vi "SetEntryJumpToMode.vi"(1 "Jump To Mode":u16(ring) items=["First", "Previous", "Next", "Last", "Item"], 3 "error in (no error)":errorcluster, 4 "Element":i16=1 min=1, 5 "VISA resource name":refnum<visa-resource-name>) -> (0 "error out":errorcluster, 2 "VISA resource name out":refnum<visa-resource-name>)   [LabVIEW 2020, in "Active Technologies AWG3000.lvlib"]
uses:
  Active Technologies AWG3000.lvlib
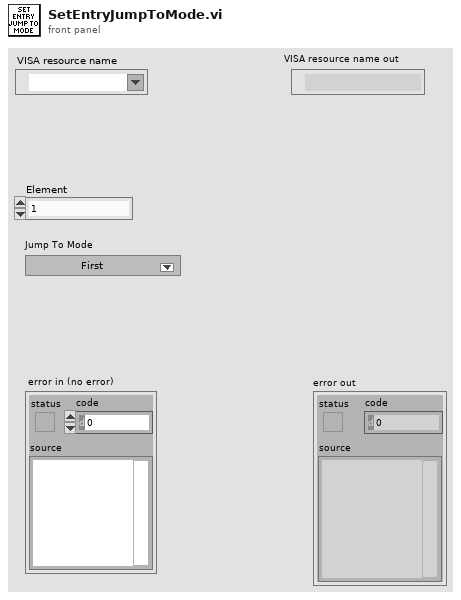
[diagram p1: front panel]
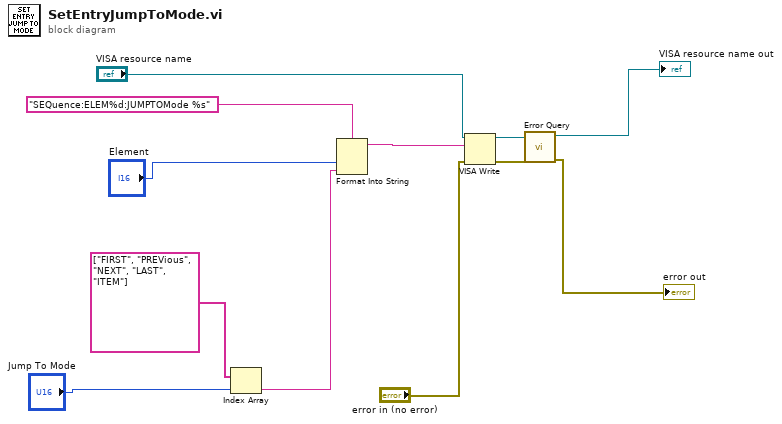
[diagram p0: block diagram]
diagram:
  n1 = Index Array(array=string[] ["FIRST", "PREVious", "NEXT", "LAST", "ITEM"], index="Jump To Mode") -> (element=w1:string)
  n2 = Format Into String(format string="SEQuence:ELEM%d:JUMPTOMode %s" ("write buffer"), "Element", w1) -> (resulting string=w4:string)  [unwired: 2 in, 1 out]
  n3 = VISA Write(VISA resource name="VISA resource name", write buffer=w4, error in (no error)="error in (no error)") -> (VISA resource name out=w9:refnum<visa-resource-name>, error out=w8:errorcluster)  [unwired: 1 out]
  n4 = call "Error Query.vi"("error in (no error)"=w8, "VISA resource name"=w9) -> ("error out"=→"error out":errorcluster, "VISA resource name out"=→"VISA resource name out":refnum<visa-resource-name>)  [unwired: 6 in, 2 out]
